vi "TestExtractScleraPlane.vi"() -> ()   [LabVIEW 2014]
uses:
  <vilib>/vision/NI_Vision_Development_Module.lvlib
panel:
  out "Source":T1(plugin-control)
  out "Result":T1(plugin-control)
  in  "File Path":path
  out "error out":errorcluster
  in  "error in":errorcluster
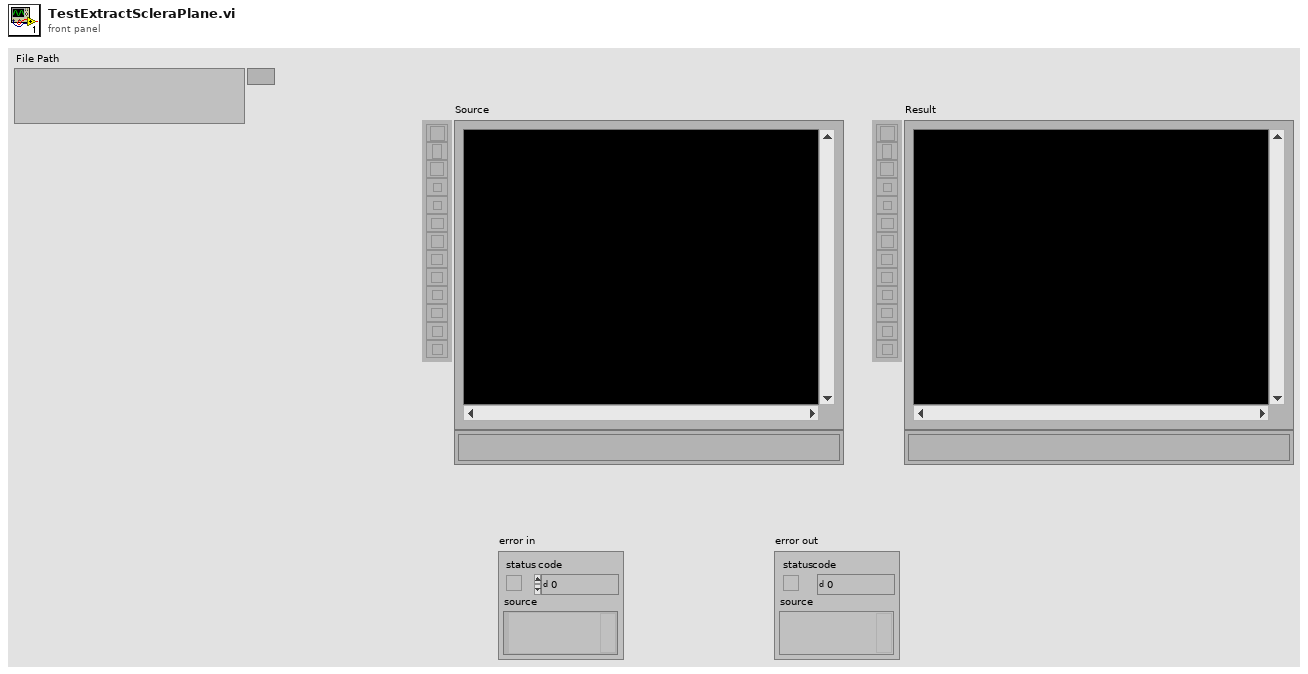
[diagram p1: front panel]
types:
  T1 = typedef "IMAQ Image.ctl" = refnum<image>
  T2 = typedef "Image Type" = u32
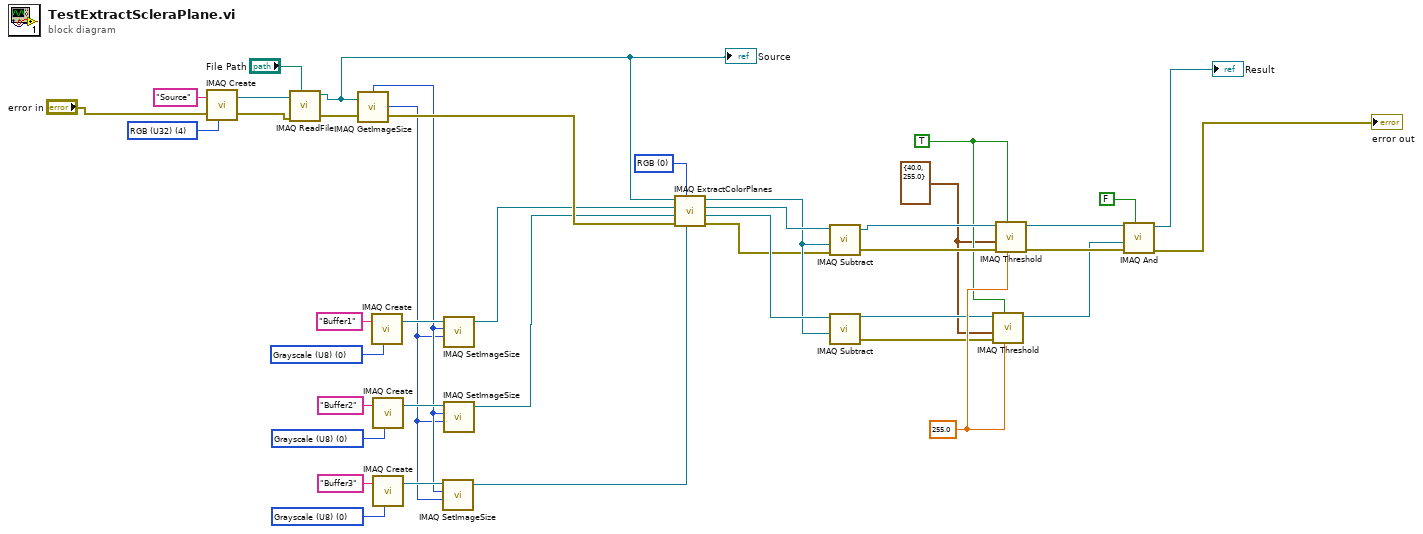
[diagram p0: block diagram]
diagram:
  w4 = cluster{"Lower value":sgl, "Upper value":sgl} {"Lower value"=40.0, "Upper value"=255.0} ("Range")
  w8 = sgl 255.0 ("Replace Value")
  w5 = TRUE ("Keep/Replace Value (Replace)")
  w13 = u16 0 items=["RGB", "HSL", "HSV", "HSI"] ("Color Mode")
  w29 = T2 0 items=["Grayscale (U8)", "Grayscale (I16)", "Grayscale (SGL)", "Complex (CSG)", "RGB (U32)", "HSL (U32)", "RGB (U64)", "Grayscale (U16)"] ("Image Type")
  w30 = T2 0 items=["Grayscale (U8)", "Grayscale (I16)", "Grayscale (SGL)", "Complex (CSG)", "RGB (U32)", "HSL (U32)", "RGB (U64)", "Grayscale (U16)"] ("Image Type")
  w31 = T2 0 items=["Grayscale (U8)", "Grayscale (I16)", "Grayscale (SGL)", "Complex (CSG)", "RGB (U32)", "HSL (U32)", "RGB (U64)", "Grayscale (U16)"] ("Image Type")
  w34 = T2 4 items=["Grayscale (U8)", "Grayscale (I16)", "Grayscale (SGL)", "Complex (CSG)", "RGB (U32)", "HSL (U32)", "RGB (U64)", "Grayscale (U16)"] ("Image Type")
  n1 = call "IMAQ Create"("Image Name"="Source", "Image Type"=w34, "error in (no error)"="error in") -> ("New Image"=w35:T1, "error out"=w32:errorcluster)  [unwired: 2 in]
  n2 = call "IMAQ ReadFile"("File Path"="File Path", "error in (no error)"=w32, "Image"=w35) -> ("error out"=w24:errorcluster, "Image Out"=w1:T1)  [unwired: 4 in, 3 out]
  "Source" <- w1
  n3 = call "IMAQ GetImageSize"("Image"=w1, "error in (no error)"=w24) -> ("Y Resolution"=w14:i32, "X Resolution"=w15:i32, "error out"=w23:errorcluster)  [unwired: 2 in]
  n4 = call "IMAQ Create"("Image Name"="Buffer1", "Image Type"=w31) -> ("New Image"=w21:T1)  [unwired: 3 in, 1 out]
  n5 = call "IMAQ Create"("Image Name"="Buffer2", "Image Type"=w30) -> ("New Image"=w19:T1)  [unwired: 3 in, 1 out]
  n6 = call "IMAQ Create"("Image Name"="Buffer3", "Image Type"=w29) -> ("New Image"=w17:T1)  [unwired: 3 in, 1 out]
  n7 = call "IMAQ SetImageSize"("Y Resolution"=w14, "X Resolution"=w15, "Image"=w17) -> ("Image Out"=w16:T1)  [unwired: 2 in, 1 out]
  n8 = call "IMAQ SetImageSize"("Y Resolution"=w14, "X Resolution"=w15, "Image"=w21) -> ("Image Out"=w20:T1)  [unwired: 2 in, 1 out]
  n9 = call "IMAQ SetImageSize"("Y Resolution"=w14, "X Resolution"=w15, "Image"=w19) -> ("Image Out"=w18:T1)  [unwired: 2 in, 1 out]
  n10 = call "IMAQ ExtractColorPlanes"("Blue or Luma or Val or Inten Plane"=w16, "Color Mode"=w13, "error in (no error)"=w23, "Green or Sat Plane"=w18, "Red or Hue Plane"=w20, "Image Src"=w1) -> ("error out"=w38:errorcluster, "Blue or Luma or Val or Inten Plane out"=w40:T1, "Green or Sat Plane out"=w41:T1, "Red or Hue Plane out"=w39:T1)  [unwired: 2 in]
  n11 = call "IMAQ Subtract"("Image Src A"=w41, "Image Src B"=w39, "error in (no error)"=w38) -> ("Image Dst Out"=w10:T1, "error out"=w9:errorcluster)  [unwired: 4 in]
  n12 = call "IMAQ Subtract"("Image Src A"=w40, "Image Src B"=w39) -> ("Image Dst Out"=w7:T1, "error out"=w6:errorcluster)  [unwired: 5 in]
  n13 = call "IMAQ Threshold"("Replace Value"=w8, "Keep/Replace Value (Replace)"=w5, "error in (no error)"=w6, "Range"=w4, "Image Src"=w7) -> ("Image Dst Out"=w3:T1)  [unwired: 5 in, 1 out]
  n14 = call "IMAQ Threshold"("Replace Value"=w8, "Keep/Replace Value (Replace)"=w5, "error in (no error)"=w9, "Range"=w4, "Image Src"=w10) -> ("error out"=w12:errorcluster, "Image Dst Out"=w11:T1)  [unwired: 5 in]
  n15 = call "IMAQ And"("And/Nand (And)"=FALSE, "error in (no error)"=w12, "Image Src B"=w3, "Image Src A"=w11) -> ("error out"=→"error out":errorcluster, "Image Dst Out"=→"Result":T1)  [unwired: 6 in]
